vi "Wait for Data Ready.vi"(8 "error in (no error)":errorcluster, 10 "Timeout (10000 ms)":u32=10000, 11 "VISA resource name":refnum<visa-resource-name>) -> (0 "error out":errorcluster, 3 "VISA resource name out":refnum<visa-resource-name>)   [LabVIEW 2020, in "Keithley 6517.lvlib"]
doc: "Read the Operation Event Registers to check whether the instrument is in idle state. \n\n<B>Note:</B>\nThis VI only supports for one trigger cycle, that is to say, it is only effective when <B>Initiation Option</B> in <B>Initiate VI</B> selects <B>Immediate</B>."
uses:
  <instrlib>/Keithley 6517/Keithley 6517.lvlib
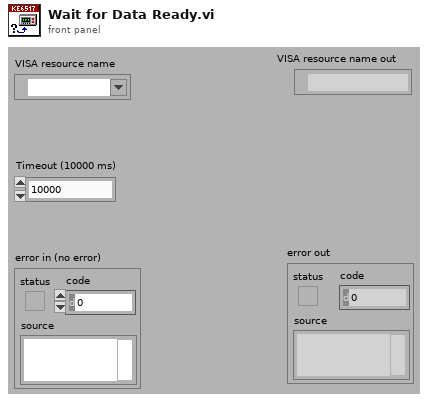
[diagram p1: front panel]
types:
  T1 = typedef "Keithley 6517.lvlib/Extended User Data.ctl" = cluster{"Instrument Model":i32}
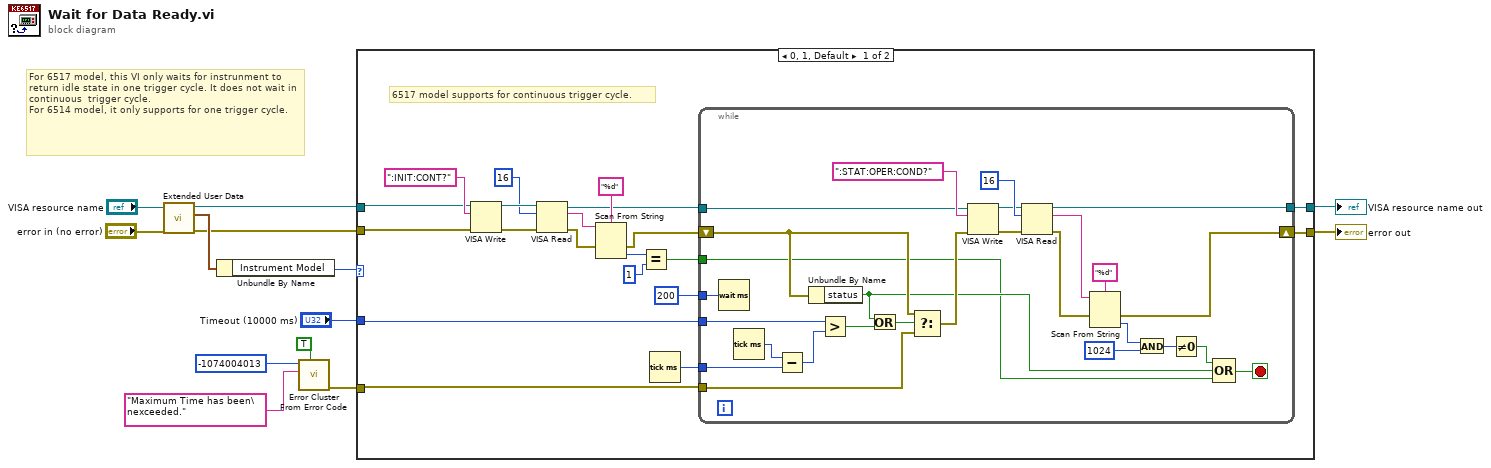
[diagram p0: block diagram]
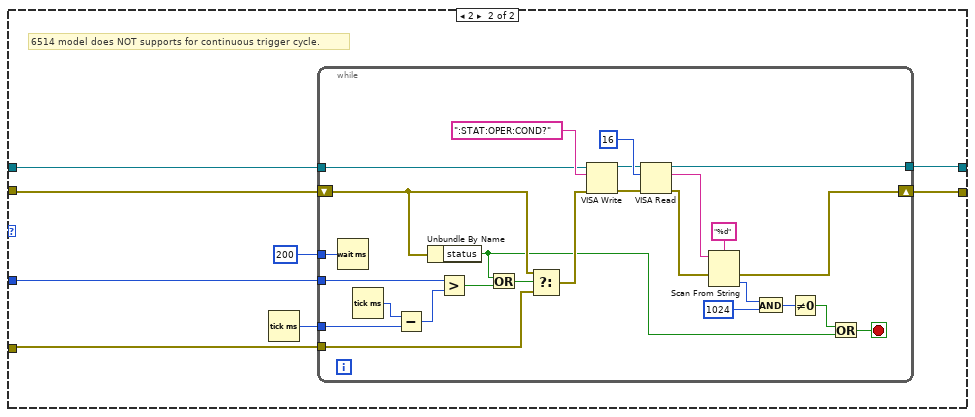
[diagram p2: hidden frame]
diagram:
  # "For 6517 model, this VI only waits for instrunment to return idle state in one trigger cycle. It does not wait in continuous  trigger cycle. \nFor 6514 model, it only supports for one trigger cycle."
  n1 = call <instrlib>:"Extended User Data.vi"("error in (no error)"="error in (no error)", "VISA resource name"="VISA resource name") -> ("error out"=w8:errorcluster, "User Data Out"=w11:T1, "VISA resource name out"=w9:refnum<visa-resource-name>)  [unwired: 7 in]
  n2 = Unbundle By Name(w11) -> ("Instrument Model"=w10:i32)
  n3 = call <vilib>:"Error Cluster From Error Code.vi"("show call chain? (False)"=TRUE, "error message (\"\")"="Maximum Time has been\nexceeded.", "error code (0)"=-1074004013) -> ("error out"=w1:errorcluster)  [unwired: 1 in, 5 out]
  n4 = case shown="0, 1, Default" w10 {
    tunnel: w9 -> [w19 w66]
    tunnel: w8 -> [w18 w63]
    tunnel: [w17 w65] -> w7
    tunnel: [w16 w64] -> w6
    tunnel: "Timeout (10000 ms)" -> [w15 w62]
    tunnel: w1 -> [w14 w61]
    frame 0, 1, Default {
      # "6517 model supports for continuous trigger cycle."
      n5 = VISA Write(VISA resource name=w19, write buffer=":INIT:CONT?", error in (no error)=w18) -> (VISA resource name out=w30:refnum<visa-resource-name>, error out=w31:errorcluster)  [unwired: 1 out]
      n6 = VISA Read(VISA resource name=w30, byte count=u32 16, error in (no error)=w31) -> (VISA resource name out=w24:refnum<visa-resource-name>, read buffer=w26:string, error out=w27:errorcluster)  [unwired: 1 out]
      n7 = Scan From String(format string="%d", input string=w26, error in=w27) -> (error out=w23:errorcluster, output 1=w22:i32)  [unwired: 2 in, 2 out]
      n8 = Equal?(x=w22, y=1) -> (x = y?=w20:bool)
      n9 = Tick Count (ms)() -> (millisecond timer value=w32:u32)
      n10 = while {
        tunnel: w24 -> [w47]
        tunnel: u32 200 ("milliseconds to wait") -> [w60]
        tunnel: w32 -> [w58]
        tunnel: w14 -> [w44]
        shift-right: [w40] -> w16
        shift-left: w23 -> [w43]
        tunnel: [w39] -> w17
        tunnel: w20 -> [w36]
        tunnel: w15 -> [w34]
        stop <- w35 stop-if-true
        n11 = Wait (ms)(milliseconds to wait=w60) -> ()  [unwired: 1 out]
        n12 = Tick Count (ms)() -> (millisecond timer value=w59:u32)
        n13 = Subtract(x=w59, y=w58) -> (x-y=w57:u32)
        n14 = Unbundle By Name(w43) -> ("status"=w38:bool)
        n15 = Greater?(x=w34, y=w57) -> (0:w46:bool)
        n16 = Or(x=w38, y=w46) -> (x .or. y?=w45:bool)
        n17 = Select(t=w43, s=w45, f=w44) -> (s? t:f=w42:errorcluster)
        n18 = VISA Write(VISA resource name=w47, write buffer=":STAT:OPER:COND?", error in (no error)=w42) -> (VISA resource name out=w49:refnum<visa-resource-name>, error out=w50:errorcluster)  [unwired: 1 out]
        n19 = VISA Read(VISA resource name=w49, byte count=u32 16, error in (no error)=w50) -> (VISA resource name out=w39:refnum<visa-resource-name>, read buffer=w56:string, error out=w41:errorcluster)  [unwired: 1 out]
        n20 = Scan From String(format string="%d", input string=w56, error in=w41) -> (error out=w40:errorcluster, output 1=w54:i32)  [unwired: 2 in, 2 out]
        n21 = And(x=w54, y=1024) -> (x .and. y?=w55:i32)
        n22 = Not Equal To 0?(x=w55) -> (x != 0?=w37:bool)
        n23 = Compound Arithmetic op=OR(w37, w38, w36) -> (w35:bool)
      }
    }
    frame 2 {
      # "6514 model does NOT supports for continuous trigger cycle."
      n24 = Tick Count (ms)() -> (millisecond timer value=w67:u32)
      n25 = while {
        tunnel: w66 -> [w80]
        tunnel: u32 200 ("milliseconds to wait") -> [w94]
        tunnel: w62 -> [w93]
        tunnel: w67 -> [w91]
        tunnel: w61 -> [w77]
        shift-right: [w73] -> w64
        shift-left: w63 -> [w76]
        tunnel: [w72] -> w65
        stop <- w71 stop-if-true
        n26 = Wait (ms)(milliseconds to wait=w94) -> ()  [unwired: 1 out]
        n27 = Tick Count (ms)() -> (millisecond timer value=w92:u32)
        n28 = Subtract(x=w92, y=w91) -> (x-y=w90:u32)
        n29 = Unbundle By Name(w76) -> ("status"=w69:bool)
        n30 = Greater?(x=w93, y=w90) -> (0:w79:bool)
        n31 = Or(x=w69, y=w79) -> (x .or. y?=w78:bool)
        n32 = Select(t=w76, s=w78, f=w77) -> (s? t:f=w75:errorcluster)
        n33 = VISA Write(VISA resource name=w80, write buffer=":STAT:OPER:COND?", error in (no error)=w75) -> (VISA resource name out=w82:refnum<visa-resource-name>, error out=w83:errorcluster)  [unwired: 1 out]
        n34 = VISA Read(VISA resource name=w82, byte count=u32 16, error in (no error)=w83) -> (VISA resource name out=w72:refnum<visa-resource-name>, read buffer=w89:string, error out=w74:errorcluster)  [unwired: 1 out]
        n35 = Scan From String(format string="%d", input string=w89, error in=w74) -> (error out=w73:errorcluster, output 1=w87:i32)  [unwired: 2 in, 2 out]
        n36 = And(x=w87, y=1024) -> (x .and. y?=w88:i32)
        n37 = Not Equal To 0?(x=w88) -> (x != 0?=w70:bool)
        n38 = Or(x=w70, y=w69) -> (x .or. y?=w71:bool)
      }
    }
  }
  "VISA resource name out" <- w7
  "error out" <- w6
